vi "File.vi"(6 "File_state":T4, 8 "error in":errorcluster caption="entrée d'erreur", 11 "Data_ini_Read":T1) -> (0 "error out":errorcluster caption="sortie d'erreur", 3 "Data_ini_Write":T1)   [LabVIEW 2020]
doc: "Read / Write INI file"
uses:
  Controls/ctrl_file_state.ctl
  Controls/ctrl_data_ini.ctl
  Controls/ctrl_ref_moteur.ctl
  Controls/ctrl_ref_camera.ctl
  <vilib>/Utility/xml.llb/Read From XML File(string).vi
  <vilib>/Utility/xml.llb/Write to XML File(string).vi
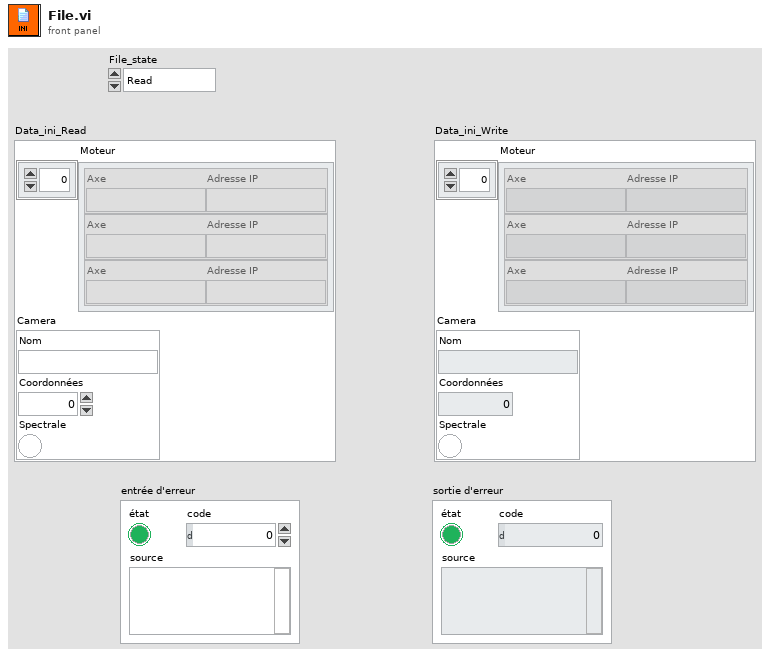
[diagram p1: front panel]
types:
  T1 = typedef "ctrl_data_ini.ctl" = cluster{"Moteur":T2[], "Camera":T3}
  T2 = typedef "ctrl_ref_moteur.ctl" = cluster{"Axe":string, "Adresse IP":string}
  T3 = typedef "ctrl_ref_camera.ctl" = cluster{"Nom":string, "Coordonnées":dbl, "Spectrale":bool}
  T4 = typedef "ctrl_file_state.ctl" = enum16{"Read", "Write"}
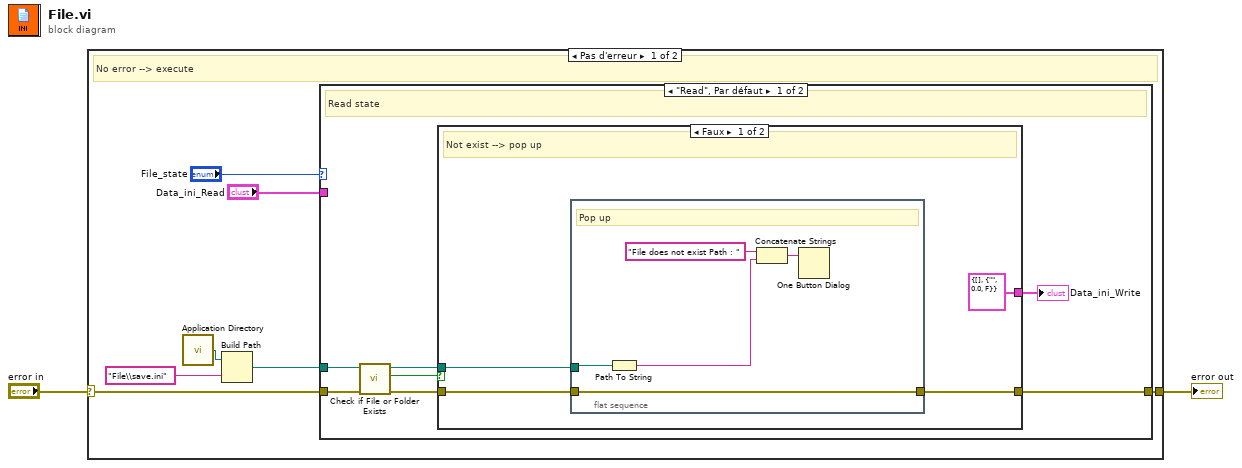
[diagram p0: block diagram]
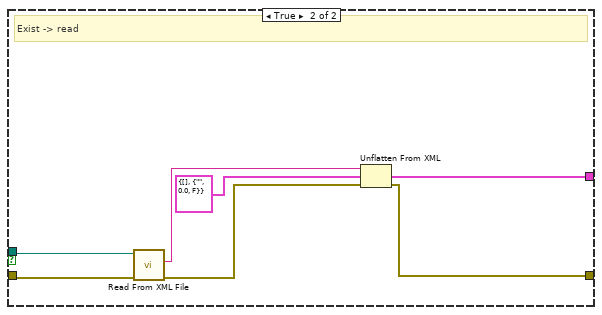
[diagram p2: hidden frame]
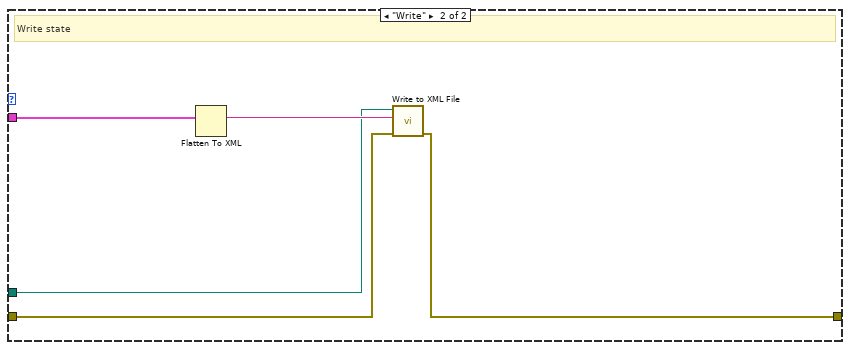
[diagram p3: hidden frame]
diagram:
  n1 = case shown="Pas d'erreur" "error in" {
    selector: "error in" -> [w7 w38]
    tunnel: [w6 w38] -> w1
    frame No Error {
      # "No error --> execute"
      n2 = call <vilib>:"Application Directory.vi"() -> ("Application Directory"=w9:path)
      n3 = Build Path(base path=w9, name or relative path="File\\save.ini") -> (appended path=w4:path)
      n4 = case shown="\"Read\", Par défaut" "File_state" {
        tunnel: w7 -> [w15 w34]
        tunnel: [w11 w33] -> w6
        tunnel: w4 -> [w16 w35]
        tunnel: "Data_ini_Read" -> [_ w37]
        frame "Read", Default {
          # "Read state"
          n5 = call <vilib>:"Check if File or Folder Exists.vi"("error in (no error)"=w15, "path"=w16) -> ("error out"=w14:errorcluster, "file or folder exists?"=w13:bool, "dup path"=w12:path)  [unwired: 7 in]
          n6 = case shown="Faux" w13 {
            tunnel: w14 -> [w20 w32]
            tunnel: w12 -> [w17 w31]
            tunnel: [w19 w27] -> w11
            tunnel: [T1 {"Moteur"=[], "Camera"={"Nom"="", "Coordonnées"=0.0, "Spectrale"=FALSE}} ("Data_ini_Write 2") w26] -> w10
            frame False {
              # "Not exist --> pop up"
              n7 = flat-sequence {
                tunnel: w20 -> [w25]
                tunnel: [w25] -> w19
                tunnel: w17 -> [w23]
                frame #0 {
                  # "Pop up"
                  n8 = Path To String(path=w23) -> (string=w22:string)
                  n9 = Concatenate Strings("File does not exist Path : " ("message"), w22) -> (w21:string)
                  n10 = One Button Dialog(message=w21) -> ()  [unwired: 1 in, 1 out]
                }
              }
            }
            frame True {
              # "Exist -> read"
              n11 = call-poly <vilib>:"Read From XML File.vi"("error in (no error)"=w32, "XML File Path"=w31) -> ("error out"=w28:errorcluster, "XML Elements"=w30:string)  [unwired: 7 in, 1 out]
              n12 = Unflatten From XML(xml string=w30, type=T1 {"Moteur"=[], "Camera"={"Nom"="", "Coordonnées"=0.0, "Spectrale"=FALSE}} ("Data_ini_Write 2"), error in (no error)=w28) -> (value=w26:T1, error out=w27:errorcluster)
            }
          }
          "Data_ini_Write" <- w10
        }
        frame "Write" {
          # "Write state"
          n13 = Flatten To XML(6:w37) -> (2:w36:string)
          n14 = call-poly <vilib>:"Write to XML File.vi"("error in (no error)"=w34, "XML Input"=w36, "XML File Path"=w35) -> ("error out"=w33:errorcluster)  [unwired: 6 in, 2 out]
        }
      }
    }
    frame Error {
      # "Error --> no execution"
    }
  }
  "error out" <- w1
